vi "GenerateILCResponseEvent.vi"(11 "ILCData":u8[](array[numeric])) -> (0 "error out":errorcluster)   [LabVIEW 2016]
panel:
  in  "User Events":T1
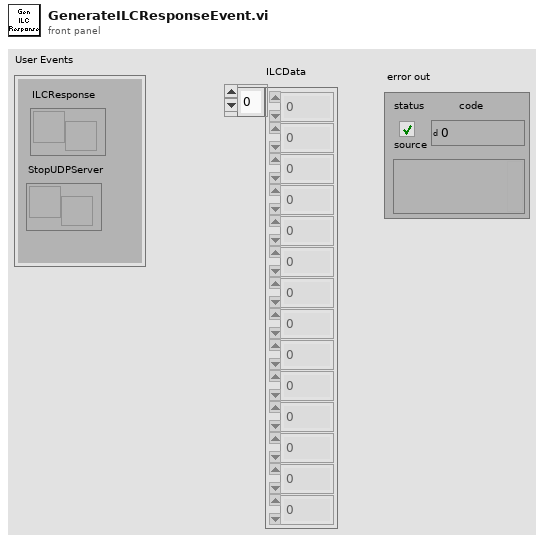
[diagram p1: front panel]
types:
  T1 = cluster{"ILCResponse":refnum<user-event>, "StopUDPServer":refnum<user-event>}
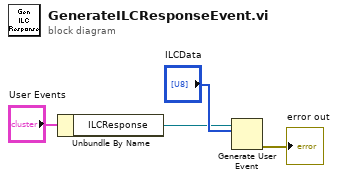
[diagram p0: block diagram]
diagram:
  n1 = Unbundle By Name("User Events") -> ("ILCResponse"=w1:refnum<user-event>)
  n2 = Generate User Event(user event=w1, event data cluster="ILCData") -> (error out=→"error out":errorcluster)  [unwired: 2 in, 1 out]
